vi "LM3Sxxxx_Comp_Config.vi"(8 "error in (no error)":errorcluster, 10 "Config Data":string[](array[string]), 11 "Interrupt Name":string) -> (0 "error out":errorcluster, 3 "Interrupt Configuration":string[](array[string]))   [LabVIEW 2011]
panel:
  in  "help":bool
  in  "Invert output":bool
  in  "Voltage reference":u32(ring)=527 items=["External pin"=0, "2.371875 V"=527, "2.26875 V"=526, "2.165625 V"=525, "2.0625"=783, "1.959375 V"=523, "1.925 V"=782, "1.85625 V"=522, "1.7875 V"=781, "1.753125 V"=521, "1.65 V"=780, "1.546875 V"=519, "1.5125 V"=779, "1.44375 V"=518, "1.375 V"=778, "1.34375 V"=515, "1.340625 V"=517, "1.2375 V"=777, "1.1 V"=776, "1.03125 V"=514, "0.9625 V"=775, "0.928125 V"=513, "0.825 V"=774, "0.6875 V"=773, "0.55 V"=772, "0.4125 V"=771, "0.275 V"=770, "0.1375 V"=769, "0 V"=768]
  in  "cancel":bool
  in  "ok":bool
  in  "Interrupt trigger":u32(ring)=8 items=["High"=16, "Low"=0, "High transition"=8, "Low transition"=4, "Both transitions"=12]
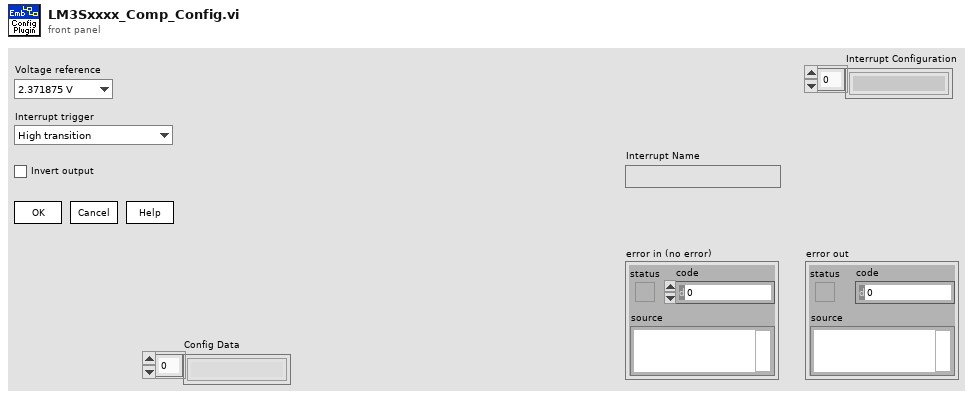
[diagram p1: front panel]
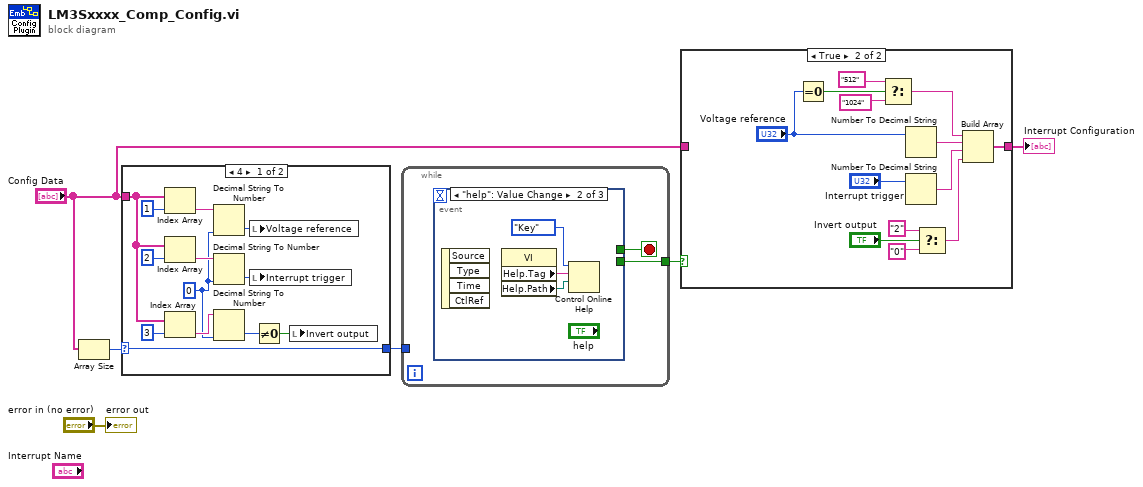
[diagram p0: block diagram]
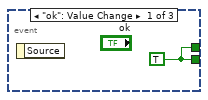
[diagram p3: hidden frame]
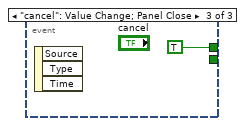
[diagram p4: hidden frame]
diagram:
  n1 = Array Size(array="Config Data") -> (size(s)=w2:i32)
  n2 = case shown="4" w2 {
    selector: w2 -> [w19 w20]
    tunnel: [w19 w20] -> w4
    tunnel: "Config Data" -> [w18 _]
    frame 4 {
      w11 = u32 0 ("default (0 I32)")
      n3 = Index Array(array=w18, index=1) -> (element=w14:string)
      n4 = Index Array(array=w18, index=2) -> (element=w13:string)
      n5 = Index Array(array=w18, index=3) -> (element=w12:string)
      n6 = Decimal String To Number(string=w14, default (0L)=w11) -> (number=w7:u32)  [unwired: 1 in, 1 out]
      n7 = Decimal String To Number(string=w13, default (0L)=w11) -> (number=w8:u32)  [unwired: 1 in, 1 out]
      n8 = Decimal String To Number(string=w12, default (0L)=w11) -> (number=w10:u32)  [unwired: 1 in, 1 out]
      n9 = local write "Voltage reference"(w7) -> ()
      n10 = local write "Interrupt trigger"(w8) -> ()
      n11 = Not Equal To 0?(x=w10) -> (x != 0?=w9:bool)
      n12 = local write "Invert output"(w9) -> ()
    }
    frame Default {
    }
  }
  n13 = while {
    tunnel: [w21] -> w5
    tunnel: w4 -> [_]
    stop <- w22 stop-if-true
    n14 = event shown="[1] \"help\": Value Change" {
      selector: _ -> [_ _ _]
      dyn-events: _ -> [_ _ _]
      timeout: _ -> [_ _ _]
      tunnel: [w23 _ TRUE] -> w22
      tunnel: [w23 _ _] -> w21
      event "ok": Value Change {
        w23 = TRUE
        n15 = event-data() -> ()  [unwired: 2 out]
      }
      event "help": Value Change {
        n16 = event-data() -> ()  [unwired: 5 out]
        n17 = property class="VI"() -> ("Help.Tag"=w24:string, "Help.Path"=w25:path)  [unwired: 2 in, 2 out]
        n18 = Control Online Help(2:w25, 3:w24, 4:enum16{"Contents", "Key", "Close"}."Key" ("Operation")) -> ()  [unwired: 1 in, 1 out]
      }
      event "cancel": Value Change; Panel Close {
        n19 = event-data() -> ()  [unwired: 4 out]
      }
    }
  }
  n20 = case shown="True" w5 {
    tunnel: [w28 w40] -> w3
    tunnel: "Config Data" -> [w28 _]
    frame False {
    }
    frame True {
      n21 = Equal To 0?(x="Voltage reference") -> (x = 0?=w32:bool)
      n22 = Select(t="512", s=w32, f="1024") -> (s? t:f=w29:string)
      n23 = Number To Decimal String(number="Voltage reference") -> (decimal integer string=w35:string)  [unwired: 1 out]
      n24 = Number To Decimal String(number="Interrupt trigger") -> (decimal integer string=w36:string)  [unwired: 1 out]
      n25 = Select(t="2", s="Invert output", f="0") -> (s? t:f=w34:string)
      n26 = Build Array(w29, w35, w36, w34) -> (w40:string[])
    }
  }
  "Interrupt Configuration" <- w3
  "error out" <- "error in (no error)"
